vi "Lab2.vi"() -> ()   [LabVIEW 2011]
panel:
  out "XY Graph":cluster{dbl[], dbl[]}(graph)
  in  "Xk":dbl
  in  "dx":dbl
  in  "X0":dbl
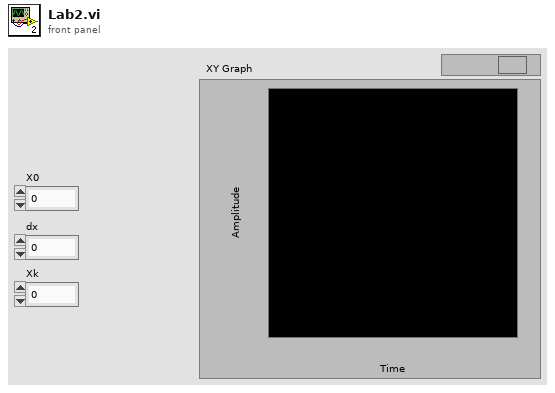
[diagram p1: front panel]
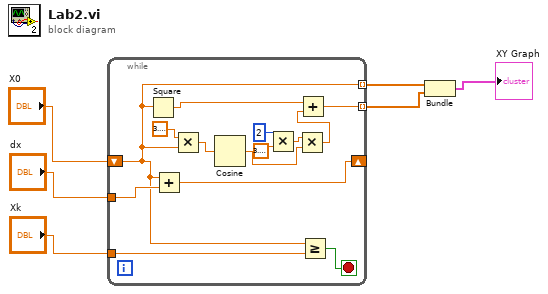
[diagram p0: block diagram]
diagram:
  n1 = while {
    shift-right: [w19] -> _
    shift-left: "X0" -> [w13]
    tunnel: "dx" -> [w20]
    tunnel: "Xk" -> [w17]
    tunnel: [w13] -> w3 mode=indexing
    tunnel: [w7] -> w2 mode=indexing
    stop <- w18 stop-if-true
    n2 = Square(x=w13) -> (x^2=w16:dbl)
    n3 = Add(x=w13, y=w20) -> (x+y=w19:dbl)
    n4 = Multiply(x=3.141592653589793, y=w13) -> (x*y=w14:dbl)
    n5 = Cosine(x=w14) -> (cos(x)=w9:dbl)
    n6 = Multiply(x=2, y=3.141592653589793) -> (x*y=w10:dbl)
    n7 = Multiply(x=w10, y=w9) -> (x*y=w8:dbl)
    n8 = Add(x=w16, y=w8) -> (x+y=w7:dbl)
    n9 = Greater Or Equal?(x=w13, y=w17) -> (x >= y?=w18:bool)
  }
  n10 = Bundle(w3, w2) -> (→"XY Graph":cluster{dbl[], dbl[]})  [unwired: 1 in]
